vi "Sensor_Values.vi"() -> ()   [LabVIEW 2019]
panel:
  in  "Wheel_D_Rotation (deg)":dbl
  in  "Wheel_C_Rotation (deg)":dbl
  in  "Wheel_B_Rotation (deg)":dbl
  in  "Wheel_A_Rotation (deg)":dbl
  in  "Drive_IMU":dbl
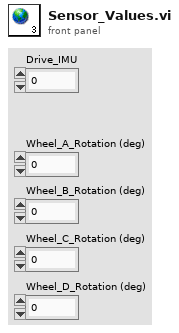
[diagram p1: front panel]
diagram:
